vi "UIinit_About.vi"(10 "Language":u32, 11 "VI输入":refnum<vi>) -> ()   [LabVIEW 2015]
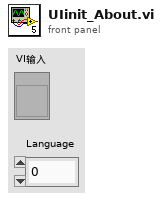
[diagram p1: front panel]
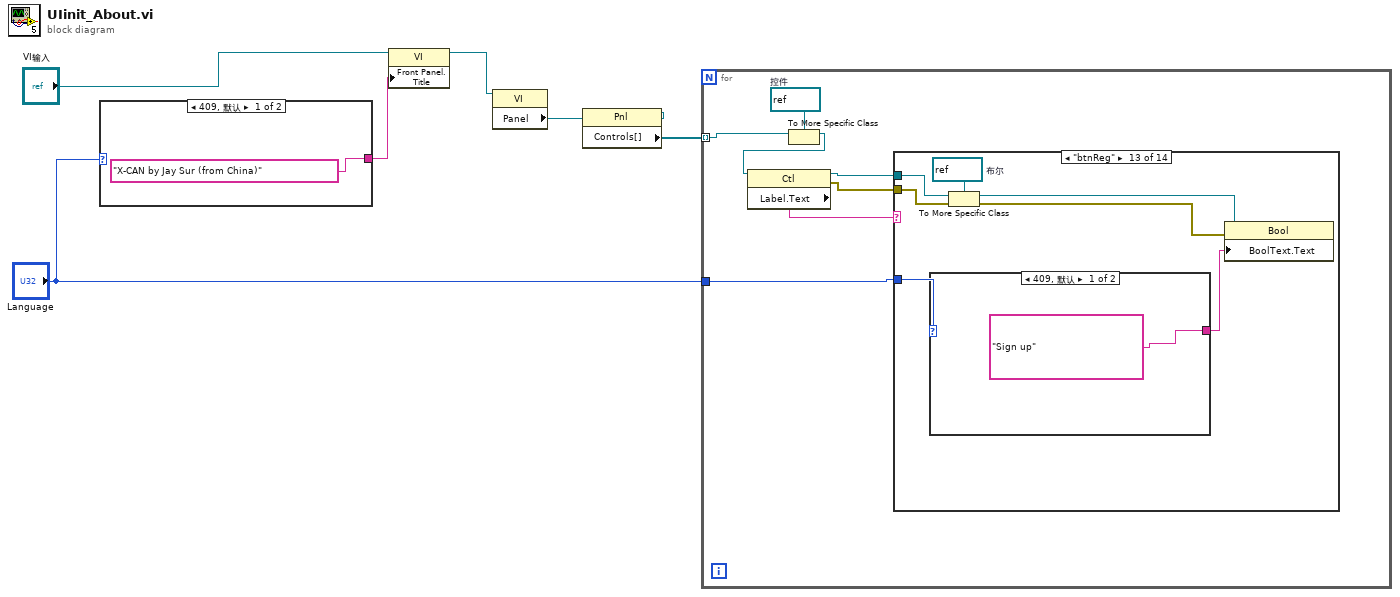
[diagram p0: block diagram]
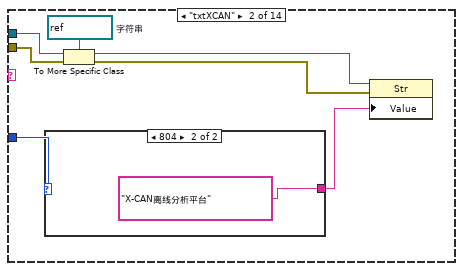
[diagram p3: hidden frame]
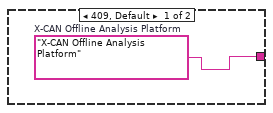
[diagram p4: hidden frame]
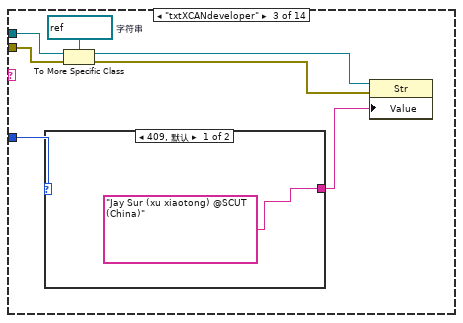
[diagram p5: hidden frame]
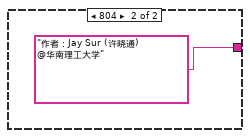
[diagram p6: hidden frame]
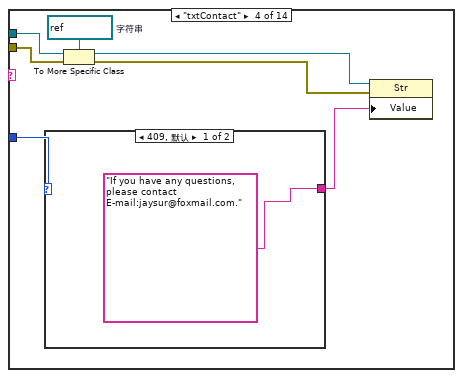
[diagram p7: hidden frame]
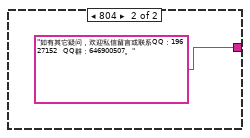
[diagram p8: hidden frame]
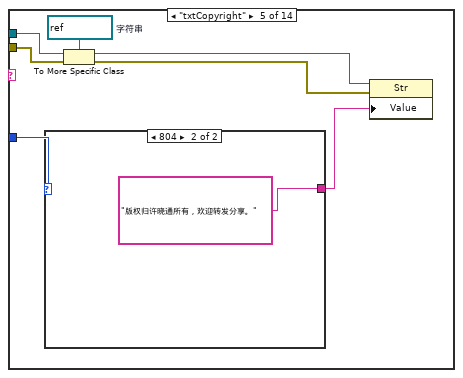
[diagram p9: hidden frame]
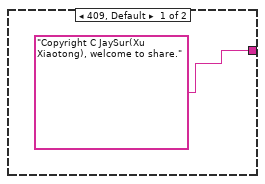
[diagram p10: hidden frame]
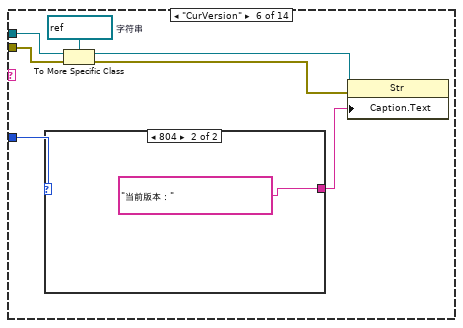
[diagram p11: hidden frame]
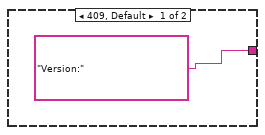
[diagram p12: hidden frame]
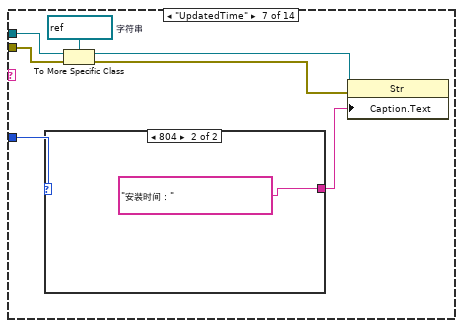
[diagram p13: hidden frame]
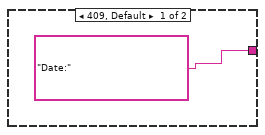
[diagram p14: hidden frame]
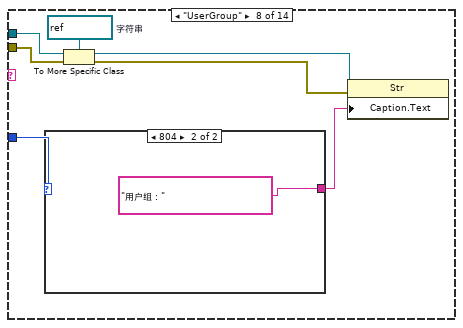
[diagram p15: hidden frame]
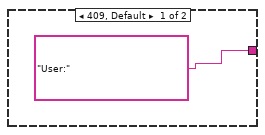
[diagram p16: hidden frame]
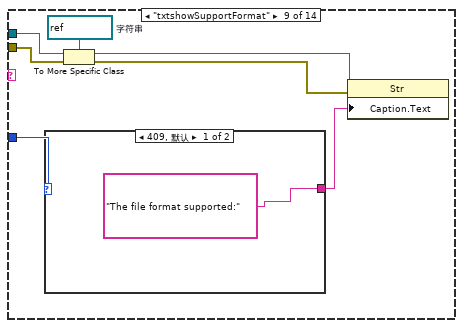
[diagram p17: hidden frame]
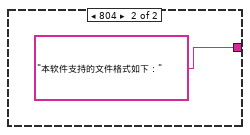
[diagram p18: hidden frame]
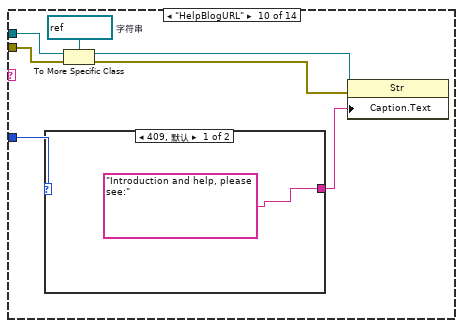
[diagram p19: hidden frame]
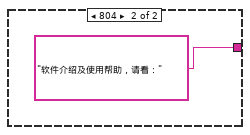
[diagram p20: hidden frame]
diagram:
  n1 = case shown="409, 默认" "Language" {
    tunnel: ["X-CAN by Jay Sur (from China)" "X-CAN by 许晓通"] -> w5
    frame 409, Default {
    }
    frame 804 {
    }
  }
  n2 = property class="VI"(reference="VI输入", "Front Panel.Title"=w5) -> (reference out=w3:refnum<vi>)  [unwired: 1 in, 1 out]
  n3 = property class="VI"(reference=w3) -> ("Panel"=w4:refnum<vi>)  [unwired: 1 in, 2 out]
  n4 = property class="Pnl"(reference=w4) -> ("Controls[]"=w2:refnum<vi>[])  [unwired: 1 in, 2 out]
  n5 = for {
    tunnel: w2 -> [w13] mode=indexing
    tunnel: "Language" -> [w10]
    w15 = refnum<vi> refnum  # 控件
    n6 = To More Specific Class(target class=w15, reference=w13) -> (specific class reference=w14:refnum<vi>)  [unwired: 1 in, 1 out]
    n7 = property class="Ctl"(reference=w14) -> (reference out=w11:refnum<vi>, error out=w9:errorcluster, "Label.Text"=w12:string)  [unwired: 1 in]
    n8 = case shown="\"btnReg\"" w12 {
      tunnel: w11 -> [_ w21 w30 w39 w48 w57 w66 w75 w84 w93 w102 w111 w120 w129]
      tunnel: w10 -> [_ w16 w25 w34 w43 w52 w61 w70 w79 w88 w97 w106 w115 w124]
      tunnel: w9 -> [_ w18 w27 w36 w45 w54 w63 w72 w81 w90 w99 w108 w117 w126]
      frame "假", Default {
      }
      frame "txtXCAN" {
        w22 = refnum<vi> refnum  # 字符串
        n9 = case shown="804" w16 {
          tunnel: [w23 "X-CAN离线分析平台"] -> w17
          frame 409, Default {
            w23 = "X-CAN Offline Analysis Platform"  # X-CAN Offline Analysis Platform
          }
          frame 804 {
          }
        }
        n10 = To More Specific Class(target class=w22, reference=w21, error in=w18) -> (specific class reference=w20:refnum<vi>, error out=w19:errorcluster)
        n11 = property class="Str"(reference=w20, error in=w19, "Value"=w17) -> ()  [unwired: 2 out]
      }
      frame "txtXCANdeveloper" {
        w31 = refnum<vi> refnum  # 字符串
        n12 = case shown="409, 默认" w25 {
          tunnel: ["Jay Sur (xu xiaotong) @SCUT (China)" "作者：Jay Sur (许晓通) @华南理工大学"] -> w26
          frame 409, Default {
          }
          frame 804 {
          }
        }
        n13 = To More Specific Class(target class=w31, reference=w30, error in=w27) -> (specific class reference=w29:refnum<vi>, error out=w28:errorcluster)
        n14 = property class="Str"(reference=w29, error in=w28, "Value"=w26) -> ()  [unwired: 2 out]
      }
      frame "txtContact" {
        w40 = refnum<vi> refnum  # 字符串
        n15 = case shown="409, 默认" w34 {
          tunnel: ["If you have any questions, please contact E-mail:jaysur@foxmail.com." "如有其它疑问，欢迎私信留言或联系QQ：19627152   QQ群：646900507。"] -> w35
          frame 409, Default {
          }
          frame 804 {
          }
        }
        n16 = To More Specific Class(target class=w40, reference=w39, error in=w36) -> (specific class reference=w38:refnum<vi>, error out=w37:errorcluster)
        n17 = property class="Str"(reference=w38, error in=w37, "Value"=w35) -> ()  [unwired: 2 out]
      }
      frame "txtCopyright" {
        w49 = refnum<vi> refnum  # 字符串
        n18 = case shown="804" w43 {
          tunnel: ["Copyright C JaySur(Xu Xiaotong), welcome to share." "版权归许晓通所有，欢迎转发分享。"] -> w44
          frame 409, Default {
          }
          frame 804 {
          }
        }
        n19 = To More Specific Class(target class=w49, reference=w48, error in=w45) -> (specific class reference=w47:refnum<vi>, error out=w46:errorcluster)
        n20 = property class="Str"(reference=w47, error in=w46, "Value"=w44) -> ()  [unwired: 2 out]
      }
      frame "CurVersion" {
        w58 = refnum<vi> refnum  # 字符串
        n21 = case shown="804" w52 {
          tunnel: ["Version:" "当前版本："] -> w53
          frame 409, Default {
          }
          frame 804 {
          }
        }
        n22 = To More Specific Class(target class=w58, reference=w57, error in=w54) -> (specific class reference=w56:refnum<vi>, error out=w55:errorcluster)
        n23 = property class="Str"(reference=w56, error in=w55, "Caption.Text"=w53) -> ()  [unwired: 2 out]
      }
      frame "UpdatedTime" {
        w67 = refnum<vi> refnum  # 字符串
        n24 = case shown="804" w61 {
          tunnel: ["Date:" "安装时间："] -> w62
          frame 409, Default {
          }
          frame 804 {
          }
        }
        n25 = To More Specific Class(target class=w67, reference=w66, error in=w63) -> (specific class reference=w65:refnum<vi>, error out=w64:errorcluster)
        n26 = property class="Str"(reference=w65, error in=w64, "Caption.Text"=w62) -> ()  [unwired: 2 out]
      }
      frame "UserGroup" {
        w76 = refnum<vi> refnum  # 字符串
        n27 = case shown="804" w70 {
          tunnel: ["User:" "用户组："] -> w71
          frame 409, Default {
          }
          frame 804 {
          }
        }
        n28 = To More Specific Class(target class=w76, reference=w75, error in=w72) -> (specific class reference=w74:refnum<vi>, error out=w73:errorcluster)
        n29 = property class="Str"(reference=w74, error in=w73, "Caption.Text"=w71) -> ()  [unwired: 2 out]
      }
      frame "txtshowSupportFormat" {
        w85 = refnum<vi> refnum  # 字符串
        n30 = case shown="409, 默认" w79 {
          tunnel: ["The file format supported:" "本软件支持的文件格式如下："] -> w80
          frame 409, Default {
          }
          frame 804 {
          }
        }
        n31 = To More Specific Class(target class=w85, reference=w84, error in=w81) -> (specific class reference=w83:refnum<vi>, error out=w82:errorcluster)
        n32 = property class="Str"(reference=w83, error in=w82, "Caption.Text"=w80) -> ()  [unwired: 2 out]
      }
      frame "HelpBlogURL" {
        w94 = refnum<vi> refnum  # 字符串
        n33 = case shown="409, 默认" w88 {
          tunnel: ["Introduction and help, please see:" "软件介绍及使用帮助，请看："] -> w89
          frame 409, Default {
          }
          frame 804 {
          }
        }
        n34 = To More Specific Class(target class=w94, reference=w93, error in=w90) -> (specific class reference=w92:refnum<vi>, error out=w91:errorcluster)
        n35 = property class="Str"(reference=w92, error in=w91, "Caption.Text"=w89) -> ()  [unwired: 2 out]
      }
      frame "GoJayWeb" {
        w103 = refnum<vi> refnum  # 布尔
        n36 = case shown="409, 默认" w97 {
          tunnel: ["My Web" "前往官网"] -> w98
          frame 409, Default {
          }
          frame 804 {
          }
        }
        n37 = To More Specific Class(target class=w103, reference=w102, error in=w99) -> (specific class reference=w101:refnum<vi>, error out=w100:errorcluster)
        n38 = property class="Bool"(reference=w101, error in=w100, "BoolText.Text"=w98) -> ()  [unwired: 2 out]
      }
      frame "btnGoBlog" {
        w112 = refnum<vi> refnum  # 布尔
        n39 = case shown="804" w106 {
          tunnel: ["My Blog" "前往博客"] -> w107
          frame 409, Default {
          }
          frame 804 {
          }
        }
        n40 = To More Specific Class(target class=w112, reference=w111, error in=w108) -> (specific class reference=w110:refnum<vi>, error out=w109:errorcluster)
        n41 = property class="Bool"(reference=w110, error in=w109, "BoolText.Text"=w107) -> ()  [unwired: 2 out]
      }
      frame "btnReg" {
        w121 = refnum<vi> refnum  # 布尔
        n42 = case shown="409, 默认" w115 {
          tunnel: ["Sign up" "注册"] -> w116
          frame 409, Default {
          }
          frame 804 {
          }
        }
        n43 = To More Specific Class(target class=w121, reference=w120, error in=w117) -> (specific class reference=w119:refnum<vi>, error out=w118:errorcluster)
        n44 = property class="Bool"(reference=w119, error in=w118, "BoolText.Text"=w116) -> ()  [unwired: 2 out]
      }
      frame "btnClose" {
        w130 = refnum<vi> refnum  # 布尔
        n45 = case shown="409, 默认" w124 {
          tunnel: ["Close" "关闭窗口"] -> w125
          frame 409, Default {
          }
          frame 804 {
          }
        }
        n46 = To More Specific Class(target class=w130, reference=w129, error in=w126) -> (specific class reference=w128:refnum<vi>, error out=w127:errorcluster)
        n47 = property class="Bool"(reference=w128, error in=w127, "BoolText.Text"=w125) -> ()  [unwired: 2 out]
      }
    }
  }
